vi "IfFileExist_DeleteFile.vi"(0 "appended path":path) -> ()   [LabVIEW 2014]
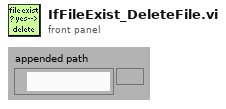
[diagram p1: front panel]
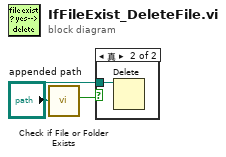
[diagram p0: block diagram]
diagram:
  n1 = call <vilib>:"Check if File or Folder Exists.vi"("path"="appended path") -> ("file or folder exists?"=w1:bool)  [unwired: 1 in, 9 out]
  n2 = case shown="真" w1 {
    tunnel: "appended path" -> [_ w3]
    frame False {
    }
    frame True {
      n3 = Delete(path (use dialog)=w3) -> ()  [unwired: 1 in, 6 out]
    }
  }
